vi "Wait On Launched Notifier Wrapper.vi"(8 "error in (no error)":errorcluster, 9 "Launch Timeout [ms]":i32=-1, 10 "Wait For Launch Completed":bool, 11 "Actor in":refnum<class "Actor.lvclass">) -> (0 "error out":errorcluster, 2 "Launch Time":timestamp, 3 "Actor out":refnum<class "Actor.lvclass">)   [LabVIEW 2015, in "Actor.lvclass"]
uses:
  Actor.lvclass
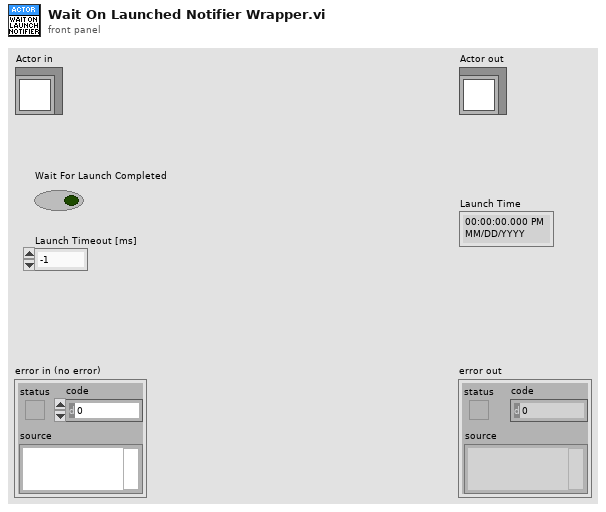
[diagram p1: front panel]
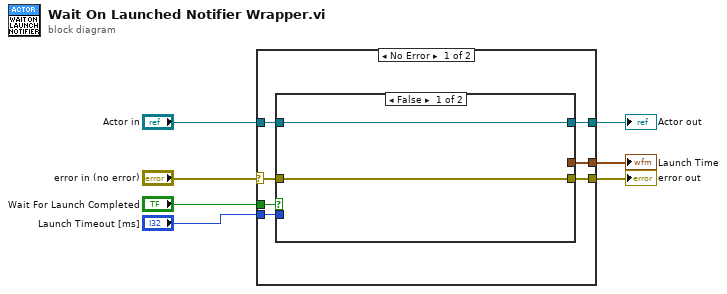
[diagram p0: block diagram]
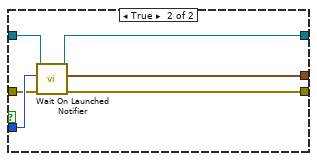
[diagram p2: hidden frame]
diagram:
  n1 = case shown="No Error" "error in (no error)" {
    selector: "error in (no error)" -> [w12 w24]
    tunnel: "Actor in" -> [w14 w23]
    tunnel: "Launch Timeout [ms]" -> [w13 _]
    tunnel: [w11 w24] -> w5
    tunnel: "Wait For Launch Completed" -> [w10 _]
    tunnel: [w9 w23] -> w4
    tunnel: [w8 _] -> w1
    frame No Error {
      n2 = case shown="False" w10 {
        tunnel: w14 -> [w15 w22]
        tunnel: w13 -> [_ w21]
        tunnel: w12 -> [w16 w20]
        tunnel: [w16 w19] -> w11
        tunnel: [w15 w18] -> w9
        tunnel: [_ w17] -> w8
        frame False {
        }
        frame True {
          n3 = call-dynamic "Wait On Launched Notifier.vi"("error in (no error)"=w20, "Launch Timeout [ms]"=w21, "Actor in"=w22) -> ("error out"=w19:errorcluster, "Launch Time"=w17:timestamp, "Actor out"=w18:refnum<class "Actor.lvclass">)  [unwired: 6 in]
        }
      }
    }
    frame Error {
    }
  }
  "error out" <- w5
  "Actor out" <- w4
  "Launch Time" <- w1
